vi "ex8-7.vi"   [LabVIEW 2009]
uses:
  <vilib>/NXT/Block Support/NXT_MessageMailbox.ctl
  <vilib>/NXT/Dual Mode Library/BT/BlueTooth_Write_String_c2.vi
types:
  T1 = typedef "NXT_MessageMailbox.ctl" = u8
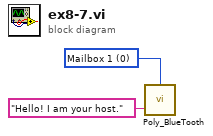
[diagram p0: block diagram]
diagram:
  w1 = T1 0 items=["Mailbox 1", "Mailbox 2", "Mailbox 3", "Mailbox 4", "Mailbox 5", "Mailbox 6", "Mailbox 7", "Mailbox 8", "Mailbox 9", "Mailbox 10"] ("Mailbox")
  n1 = call-poly <vilib>:"Poly_BlueTooth.vi"("Message"="Hello! I am your host.", "Mailbox"=w1) -> ()  [unwired: 2 in, 1 out]
